vi "FlatToRichniswitch_grpc_InitWithOptionsResponse.vi"(5 "OutputClusterType":T1, 11 "InputCluster":T3) -> (3 "OutputCluster":T1)   [LabVIEW 2021, in "NI Switch_client.lvlib"]
uses:
  NI Switch_client.lvlib
  niswitch_grpc_InitWithOptionsResponse_Flat.ctl
  nidevice_grpc_Session_Flat.ctl
  niswitch_grpc_InitWithOptionsResponse.ctl
  nidevice_grpc_Session.ctl
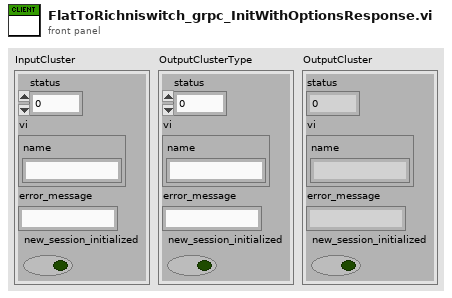
[diagram p1: front panel]
types:
  T1 = typedef "NI Switch_client.lvlib/niswitch_grpc_InitWithOptionsResponse.ctl" = cluster{"status":i32, "vi":T2, "error_message":string, "new_session_initialized":bool}
  T2 = typedef "NI Switch_client.lvlib/nidevice_grpc_Session.ctl" = cluster{"name":string}
  T3 = typedef "NI Switch_client.lvlib/niswitch_grpc_InitWithOptionsResponse_Flat.ctl" = cluster{"status":i32, "vi":T4, "error_message":string, "new_session_initialized":bool}
  T4 = typedef "NI Switch_client.lvlib/nidevice_grpc_Session_Flat.ctl" = cluster{"name":string}
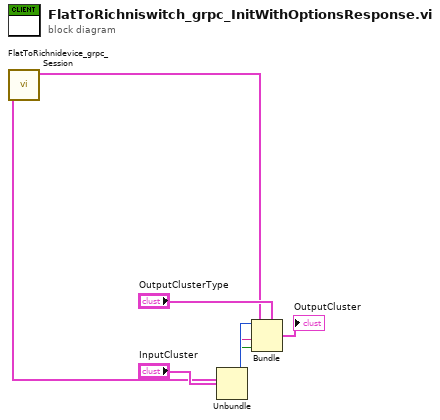
[diagram p0: block diagram]
diagram:
  n1 = Unbundle "Unbundle"("InputCluster") -> ("status"=w5:i32, "vi"=w4:T4, "error_message"=w2:string, "new_session_initialized"=w1:bool)
  n2 = call "FlatToRichnidevice_grpc_Session.vi"("InputCluster"=w4) -> ("OutputCluster"=w3:T2)  [unwired: 10 in]
  n3 = Bundle "Bundle"(cluster="OutputClusterType", "status"=w5, "vi"=w3, "error_message"=w2, "new_session_initialized"=w1) -> (→"OutputCluster":T1)
